vi "Strip UTF8 Byte Order Mark (if present).vi"(11 "Text in":string) -> (2 "Mark was stripped":bool, 3 "Possible Byte Order Mark Stripped":string)   [LabVIEW 2021, in "json.facade.lvlib"]
doc: "Removes any Byte Order Mark for UTF-8 that an external editor may have added."
uses:
  json.facade.lvlib
  jsontext/JSONtext.lvlib
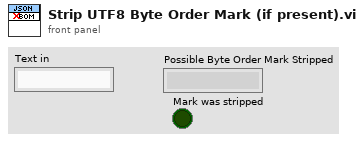
[diagram p1: front panel]
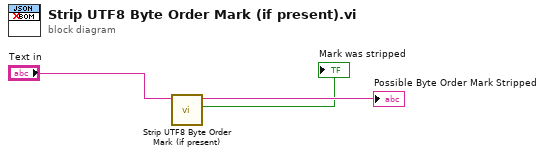
[diagram p0: block diagram]
diagram:
  n1 = call "Strip UTF8 Byte Order Mark (if present).vi"("Text in"="Text in") -> ("Mark was stripped"=→"Mark was stripped":bool, "Possible Byte Order Mark Stripped"=→"Possible Byte Order Mark Stripped":string)  [unwired: 9 in]
